vi "Wrt_Digital_OP.vi"(8 "Error In":errorcluster, 10 "Plants_Digital_OP":T4 {"Channel No" items=["7"=7, "11"=11, "12"=12, "13"=13, "15"=15, "16"=16, "18"=18, "29"=29, "32"=32, "33"=33, "35"=35, "36"=36, "37"=37, "38"=38, "40"=40]}, 11 "Read_WriteIN":T1={"Time Table"=[{"Set Time"=0.0, "Control"=enum."Time", "Duration[S]"=3.0, "Liter"=0.0, "Plant Name."="", "Watered"=FALSE, "Su"=FALSE, "Mo"=FALSE, "Tu"=FALSE, "We"=FALSE, "Th"=FALSE, "Fr"=FALSE, "Sa"=FALSE}, {"Set Time"=0.0, "Control"=enum."Time", "Duration[S]"=5.0, "Liter"=0.0, "Plant Name."="", "Watered"=FALSE, "Su"=FALSE, "Mo"=FALSE, "Tu"=FALSE, "We"=FALSE, "Th"=FALSE, "Fr"=FALSE, "Sa"=FALSE}, {"Set Time"=0.0, "Control"=enum."Time", "Duration[S]"=5.0, "Liter"=0.0, "Plant Name."="", "Watered"=FALSE, "Su"=FALSE, "Mo"=FALSE, "Tu"=FALSE, "We"=FALSE, "Th"=FALSE, "Fr"=FALSE, "Sa"=FALSE}], "Plants_Digital_OP"=[], "delta_ms_w_Index"={"delta_ms"=[], "Index"=[], "RunArray"=[]}, "TimeOutInfo"={"Timeout"=0, "ValveCTR"={"State"=enum."Open Valve", "Channel No"=0, "Duration[S]"=0.0}, "Index"=0}, "LoopName"=""} {"TimeOutInfo"."ValveCTR"."Channel No" items=["7"=7, "11"=11, "12"=12, "13"=13, "15"=15, "16"=16, "18"=18, "29"=29, "32"=32, "33"=33, "35"=35, "36"=36, "37"=37, "38"=38, "40"=40]; "delta_ms_w_Index"."RunArray"."Channel No" items=["7"=7, "11"=11, "12"=12, "13"=13, "15"=15, "16"=16, "18"=18, "29"=29, "32"=32, "33"=33, "35"=35, "36"=36, "37"=37, "38"=38, "40"=40]; "Plants_Digital_OP"."Channel No" items=["7"=7, "11"=11, "12"=12, "13"=13, "15"=15, "16"=16, "18"=18, "29"=29, "32"=32, "33"=33, "35"=35, "36"=36, "37"=37, "38"=38, "40"=40]; "Time Table"."Liter" min=0.0; "Time Table"."Set Time" format="%<%.H:%M:%S>T"; "Time Table"."Duration[S]" min=0.0}) -> (0 "Error Out":errorcluster, 3 "Read_WriteIOUT":T1={"Time Table"=[{"Set Time"=0.0, "Control"=enum."Time", "Duration[S]"=3.0, "Liter"=0.0, "Plant Name."="", "Watered"=FALSE, "Su"=FALSE, "Mo"=FALSE, "Tu"=FALSE, "We"=FALSE, "Th"=FALSE, "Fr"=FALSE, "Sa"=FALSE}, {"Set Time"=0.0, "Control"=enum."Time", "Duration[S]"=5.0, "Liter"=0.0, "Plant Name."="", "Watered"=FALSE, "Su"=FALSE, "Mo"=FALSE, "Tu"=FALSE, "We"=FALSE, "Th"=FALSE, "Fr"=FALSE, "Sa"=FALSE}, {"Set Time"=0.0, "Control"=enum."Time", "Duration[S]"=5.0, "Liter"=0.0, "Plant Name."="", "Watered"=FALSE, "Su"=FALSE, "Mo"=FALSE, "Tu"=FALSE, "We"=FALSE, "Th"=FALSE, "Fr"=FALSE, "Sa"=FALSE}], "Plants_Digital_OP"=[], "delta_ms_w_Index"={"delta_ms"=[], "Index"=[], "RunArray"=[]}, "TimeOutInfo"={"Timeout"=0, "ValveCTR"={"State"=enum."Open Valve", "Channel No"=0, "Duration[S]"=0.0}, "Index"=0}, "LoopName"=""} {"TimeOutInfo"."ValveCTR"."Channel No" items=["7"=7, "11"=11, "12"=12, "13"=13, "15"=15, "16"=16, "18"=18, "29"=29, "32"=32, "33"=33, "35"=35, "36"=36, "37"=37, "38"=38, "40"=40]; "delta_ms_w_Index"."RunArray"."Channel No" items=["7"=7, "11"=11, "12"=12, "13"=13, "15"=15, "16"=16, "18"=18, "29"=29, "32"=32, "33"=33, "35"=35, "36"=36, "37"=37, "38"=38, "40"=40]; "Plants_Digital_OP"."Channel No" items=["7"=7, "11"=11, "12"=12, "13"=13, "15"=15, "16"=16, "18"=18, "29"=29, "32"=32, "33"=33, "35"=35, "36"=36, "37"=37, "38"=38, "40"=40]; "Time Table"."Liter" min=0.0; "Time Table"."Set Time" format="%<%.H:%M:%S>T"; "Time Table"."Duration[S]" min=0.0})   [LabVIEW 2014, in "TimeBasedProd.lvlib"]
uses:
  TimeBasedProd.lvlib
  TypeDef/Plant_OP_Map.ctl
  TypeDef/Plant_OP_Map_CTR.ctl
  ValveCTRL/TypeDef/CHs_List.ctl
  TypeDef/Read_Write.ctl
  TimeTable/TypeDef/Time_Table.ctl
  TimeTable/TypeDef/Time_Table_CTR.ctl
  TypeDef/TimeOutInfo.ctl
  ValveCTRL/TypeDef/Queue_Cluster.ctl
  ValveCTRL/TypeDef/States_Enum.ctl
  TypeDef/UpdateTimeOutinfo.ctl
  <vilib>/Utility/file.llb/Write To Spreadsheet File (string).vi
  ValveCTRL/ValveCTRL.lvlib
panel:
  # "Watering Days"
  # "Watering Days"
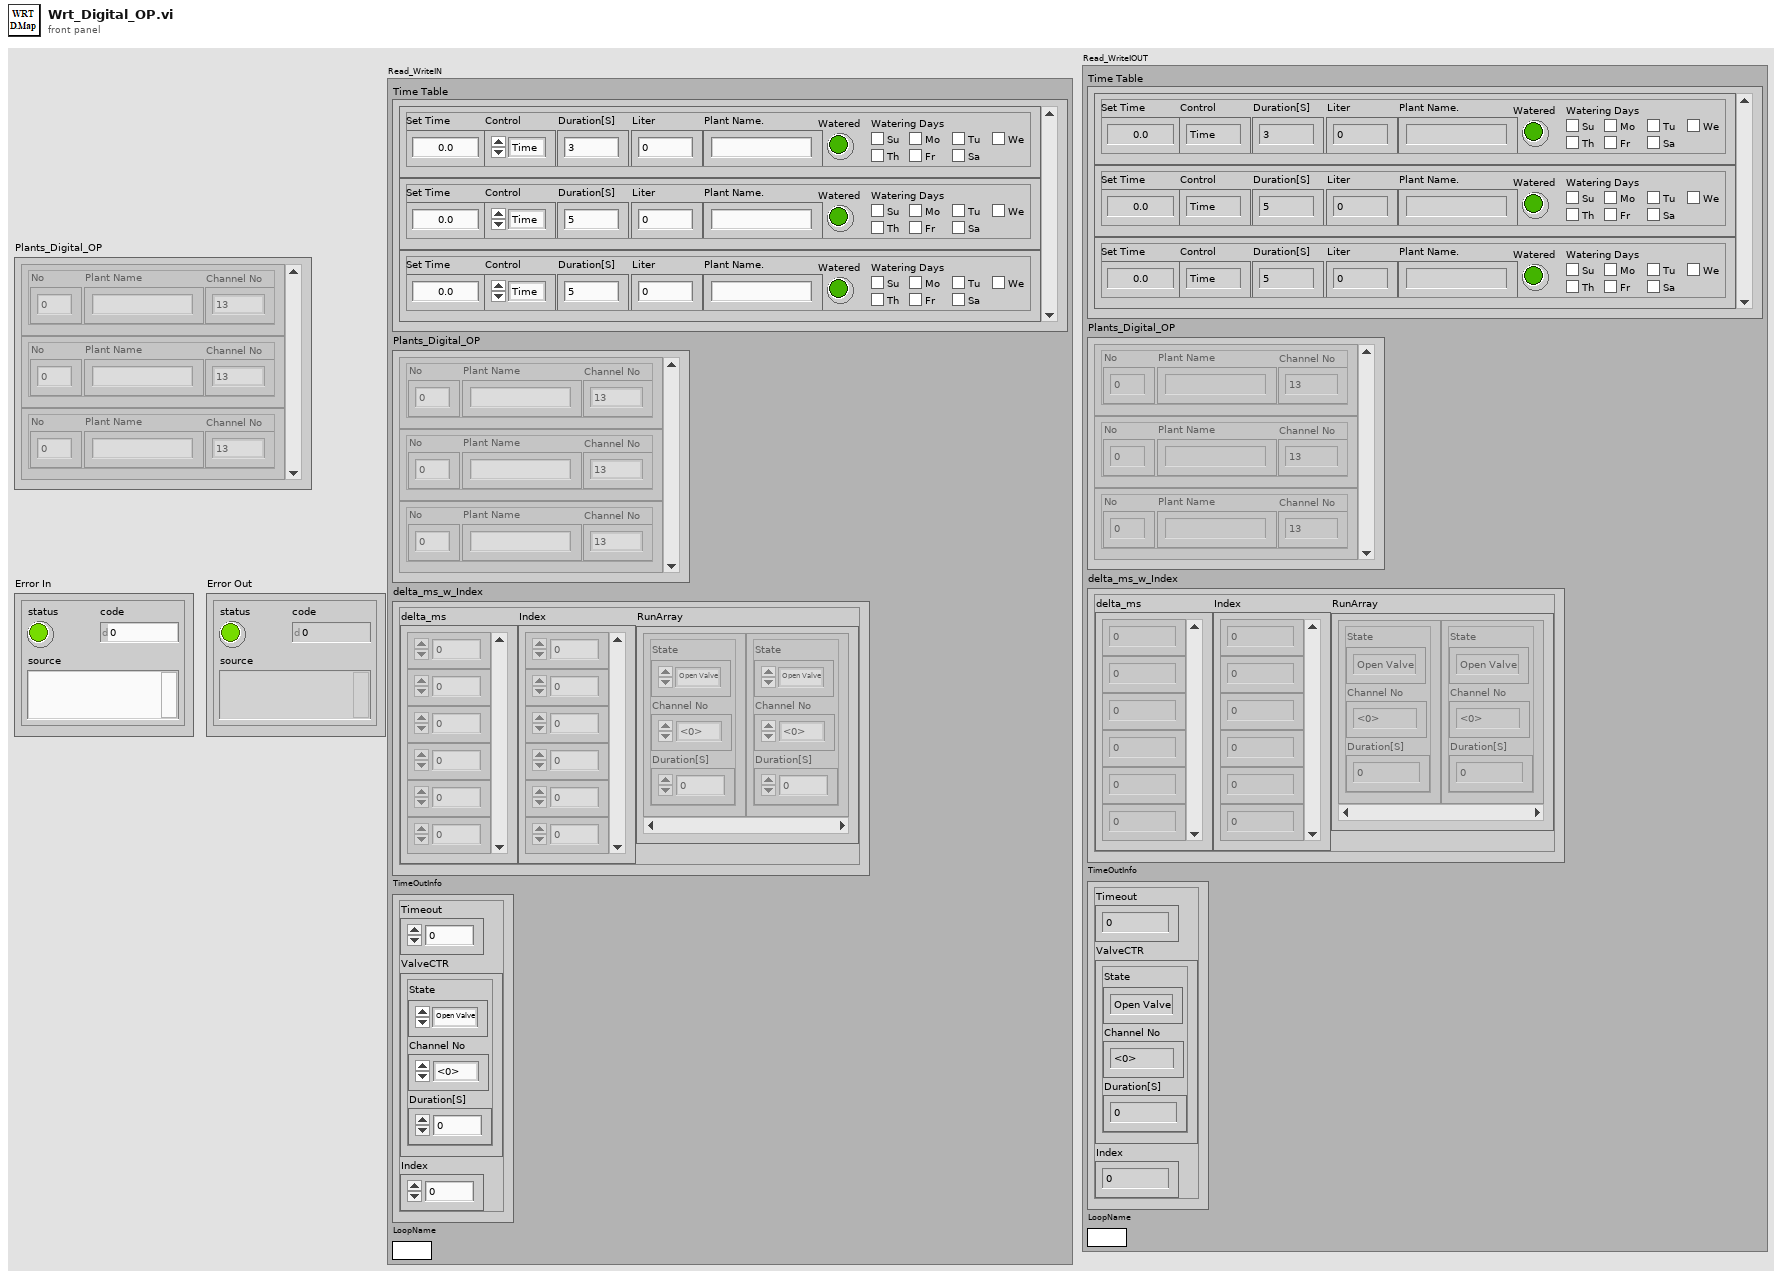
[diagram p1: front panel]
types:
  T1 = typedef "TimeBasedProd.lvlib/Read_Write.ctl" = cluster{"Time Table":T2, "Plants_Digital_OP":T4, "delta_ms_w_Index":T7, "TimeOutInfo":T10, "LoopName":string}
  T2 = typedef "TimeBasedProd.lvlib/Time_Table.ctl" = T3[]
  T3 = typedef "TimeBasedProd.lvlib/Time_Table_CTR.ctl" = cluster{"Set Time":dbl, "Control":enum16{"Time", "Flow"}, "Duration[S]":dbl, "Liter":dbl, "Plant Name.":string, "Watered":bool, "Su":bool, "Mo":bool, "Tu":bool, "We":bool, "Th":bool, "Fr":bool, "Sa":bool}
  T4 = typedef "TimeBasedProd.lvlib/Plant_OP_Map.ctl" = T5[]
  T5 = typedef "TimeBasedProd.lvlib/Plant_OP_Map_CTR.ctl" = cluster{"No":u8, "Plant Name":string, "Channel No":T6}
  T6 = typedef "ValveCTRL.lvlib/CHs_List.ctl" = u8
  T7 = typedef "TimeBasedProd.lvlib/TimeOutInfo.ctl" = cluster{"delta_ms":i32[], "Index":i32[], "RunArray":T8[]}
  T8 = typedef "ValveCTRL.lvlib/Queue_Cluster.ctl" = cluster{"State":T9, "Channel No":T6, "Duration[S]":dbl}
  T9 = typedef "ValveCTRL.lvlib/States_Enum.ctl" = enum16{"Open Pump", "Open Valve", "Wait Valve", "Close Pump", "Close Valve", "Save State", "StopLoop"}
  T10 = typedef "TimeBasedProd.lvlib/UpdateTimeOutinfo.ctl" = cluster{"Timeout":i32, "ValveCTR":T8, "Index":i32}
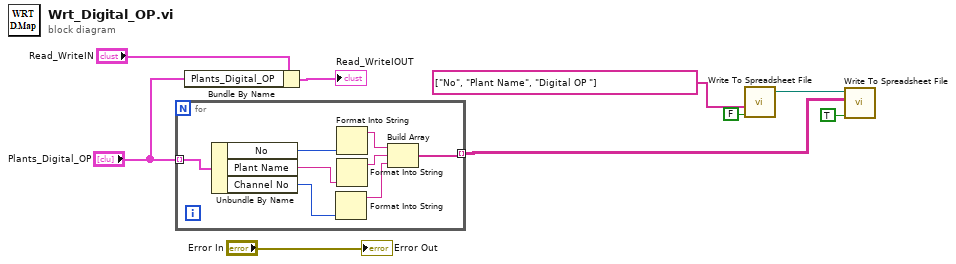
[diagram p0: block diagram]
diagram:
  n1 = for {
    tunnel: "Plants_Digital_OP" -> [w17] mode=indexing
    tunnel: [w12] -> w9 mode=indexing
    n2 = Unbundle By Name(w17) -> ("No"=w16:u8, "Plant Name"=w13:string, "Channel No"=w11:T6)
    n3 = Format Into String(w11) -> (resulting string=w10:string)  [unwired: 3 in, 1 out]
    n4 = Format Into String(w16) -> (resulting string=w15:string)  [unwired: 3 in, 1 out]
    n5 = Format Into String(w13) -> (resulting string=w14:string)  [unwired: 3 in, 1 out]
    n6 = Build Array(w15, w14, w10) -> (w12:string[])
  }
  n7 = Bundle By Name(cluster="Read_WriteIN", "Plants_Digital_OP"="Plants_Digital_OP") -> (→"Read_WriteIOUT":T1)
  n8 = call-poly <vilib>:"Write To Spreadsheet File.vi"("append to file? (new file:F)"=FALSE, "1D data"=string[] ["No", "Plant Name", "Digital OP "]) -> ("new file path (Not A Path if cancelled)"=w7:path)  [unwired: 6 in]
  n9 = call-poly <vilib>:"Write To Spreadsheet File.vi"("append to file? (new file:F)"=TRUE, "2D data"=w9, "file path (dialog if empty)"=w7) -> ()  [unwired: 5 in, 1 out]
  "Error Out" <- "Error In"
